vi "Omron TCP FINS-Command Frame.vi"(8 "error in":errorcluster, 10 "FINS Command Frame":T3, 11 "Buffer Data In":T1) -> (0 "error out":errorcluster, 3 "Buffer Data Out":T1)   [LabVIEW 2016]
uses:
  Data Def/Omron TCP FINS-FINS Command Frame.ctl
  Data Def/Omron TCP FINS-Command Code.ctl
  Data Def/Omron TCP FINS-Buffer Data.ctl
  Data Def/Omron TCP FINS-Memory Area Read Data.ctl
  Data Def/Omron TCP FINS-Memory Area Write Data.ctl
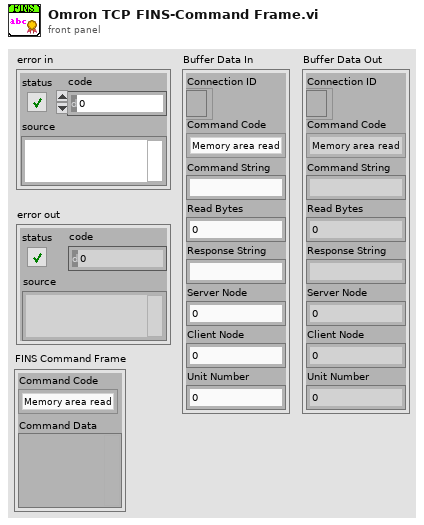
[diagram p1: front panel]
types:
  T1 = typedef "Omron TCP FINS-Buffer Data.ctl" = cluster{"Connection ID":refnum<k5>, "Command Code":T2, "Command String":string, "Read Bytes":i32, "Response String":string, "Server Node":u8, "Client Node":u8, "Unit Number":u8}
  T2 = typedef "Omron TCP FINS-Command Code.ctl" = enum16{"Memory area read", "Memory area write"}
  T3 = typedef "Omron TCP FINS-FINS Command Frame.ctl" = cluster{"Command Code":T2, "Command Data":variant}
  T4 = typedef "Omron TCP FINS-Memory Area Read Data.ctl" = cluster{"I/O Memory Address":u8, "Beginning Address":u16, "No. Of Items":u16}
  T5 = typedef "Omron TCP FINS-Memory Area Write Data.ctl" = cluster{"I/O Memory Address":u8, "Beginning Address":u16, "Data":i16[]}
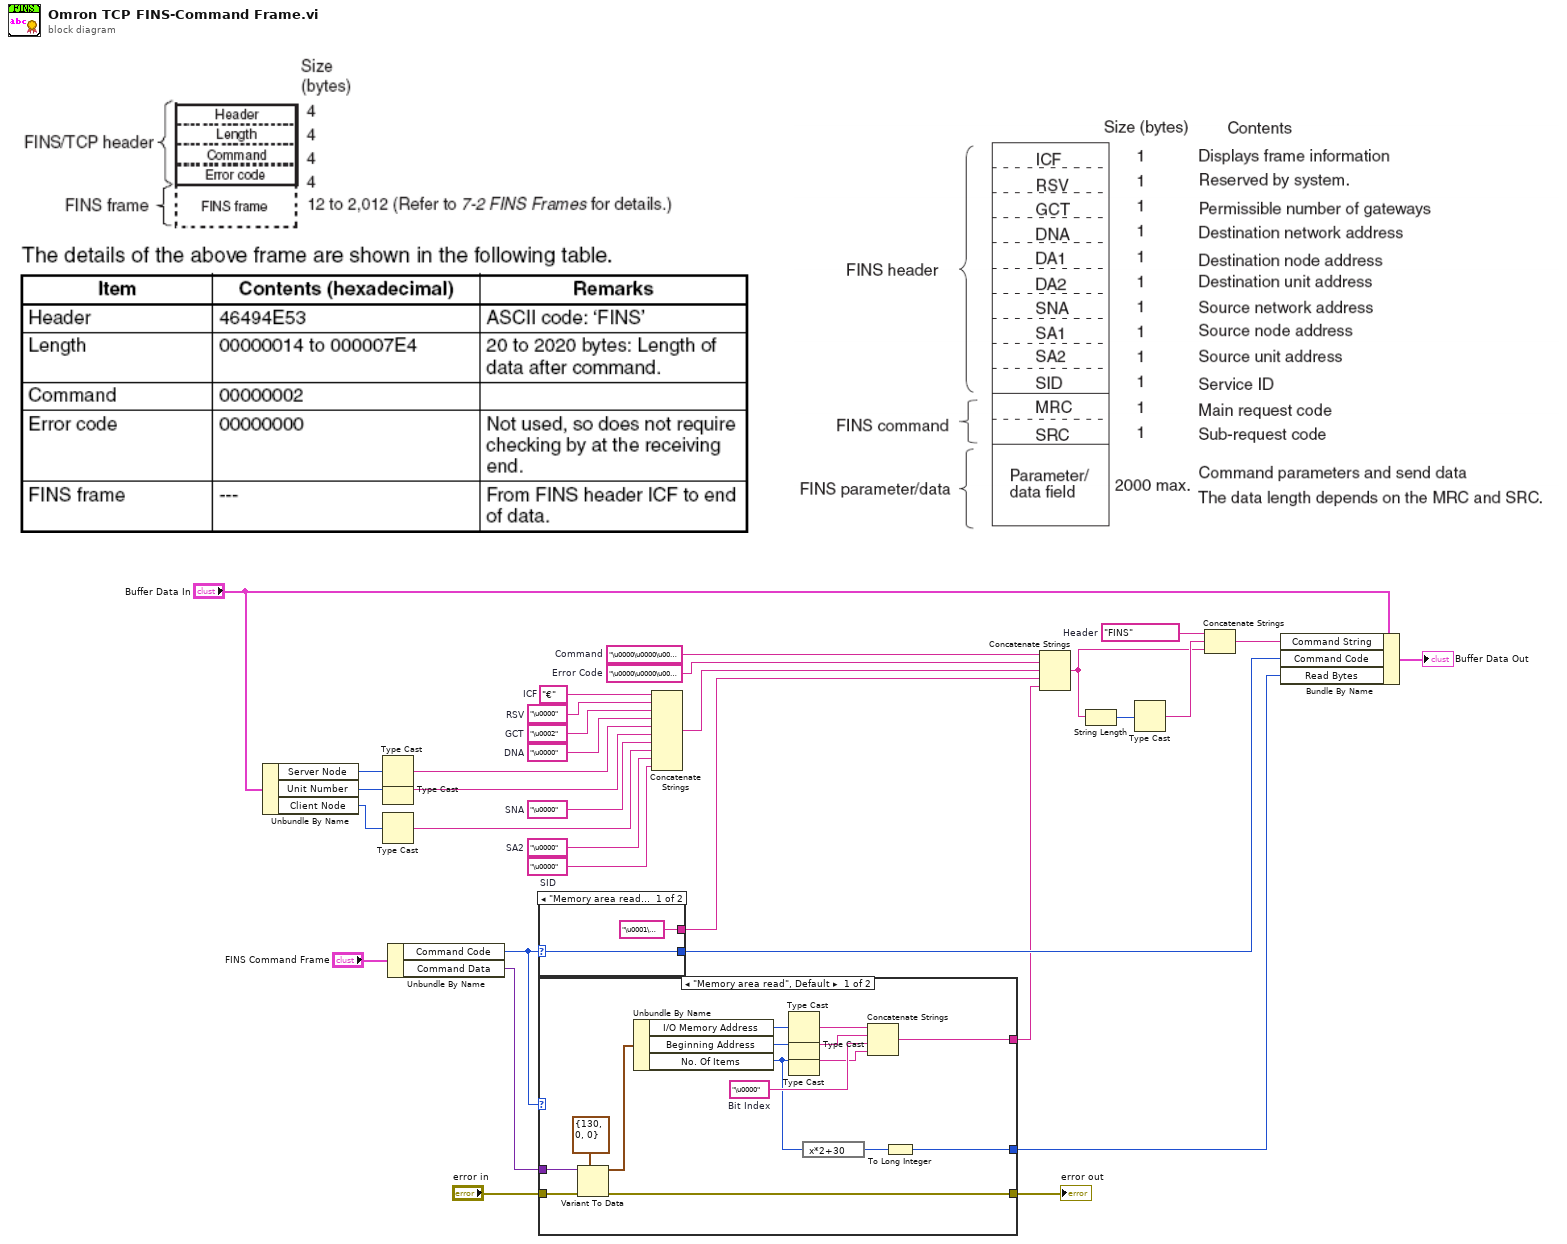
[diagram p0: block diagram]
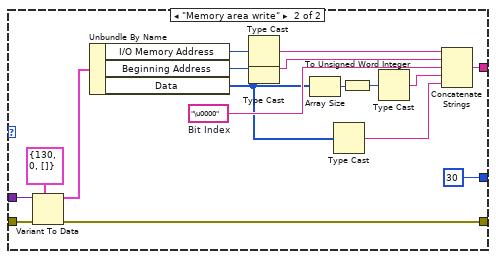
[diagram p2: hidden frame]
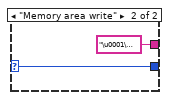
[diagram p3: hidden frame]
diagram:
  w18 = "\u0000\u0000\u0000\u0000"  # Error Code
  w19 = "\u0000\u0000\u0000\u0002"  # Command
  w20 = "\u0000"  # SID
  w21 = "\u0000"  # SA2
  w22 = "\u0000"  # SNA
  w23 = "\u0000"  # DNA
  w24 = "\u0002"  # GCT
  w25 = "\u0000"  # RSV
  w26 = "€"  # ICF
  w3 = "FINS"  # Header
  n1 = Unbundle By Name("Buffer Data In") -> ("Server Node"=w15:u8, "Unit Number"=w13:u8, "Client Node"=w11:u8)
  n2 = Type Cast(x=w15) -> (*(type *) &x=w14:string)  [unwired: 1 in]
  n3 = Type Cast(x=w13) -> (*(type *) &x=w12:string)  [unwired: 1 in]
  n4 = Type Cast(x=w11) -> (*(type *) &x=w10:string)  [unwired: 1 in]
  n5 = Unbundle By Name("FINS Command Frame") -> ("Command Code"=w32:T2, "Command Data"=w31:variant)
  n6 = case shown="\"Memory area read\", Default" w32 {
    selector: w32 -> [w33 w35]
    tunnel: ["\u0001\u0001" ("Command code") "\u0001\u0002" ("Command code")] -> w8
    tunnel: [w33 w35] -> w28
    frame "Memory area read", Default {
    }
    frame "Memory area write" {
    }
  }
  n7 = case shown="\"Memory area read\", Default" w32 {
    tunnel: w31 -> [w50 w67]
    tunnel: "error in" -> [w51 w68]
    tunnel: [w47 w65] -> w29
    tunnel: [w40 w64] -> w7
    tunnel: [w37 30 ("No. Of Items")] -> w27
    frame "Memory area read", Default {
      w42 = "\u0000"  # Bit Index
      n8 = Variant To Data(error in=w51, type=T4 {"I/O Memory Address"=130, "Beginning Address"=0, "No. Of Items"=0} ("Memory Area Read Data"), Variant=w50) -> (data=w48:T4, error out=w47:errorcluster)
      n9 = Unbundle By Name(w48) -> ("I/O Memory Address"=w46:u8, "Beginning Address"=w45:u16, "No. Of Items"=w39:u16)
      n10 = Type Cast(x=w46) -> (*(type *) &x=w44:string)  [unwired: 1 in]
      n11 = Type Cast(x=w45) -> (*(type *) &x=w43:string)  [unwired: 1 in]
      n12 = Type Cast(x=w39) -> (*(type *) &x=w41:string)  [unwired: 1 in]
      n13 = expression code="x*2+30"(w39) -> (w38:u16)
      n14 = Concatenate Strings(w44, w43, w42, w41) -> (w40:string)
      n15 = To Long Integer(number=w38) -> (32bit integer=w37:i32)
    }
    frame "Memory area write" {
      w57 = "\u0000"  # Bit Index
      n16 = Variant To Data(error in=w68, type=T5 {"I/O Memory Address"=130, "Beginning Address"=0, "Data"=[]} ("Memory Area Write Data"), Variant=w67) -> (data=w66:T5, error out=w65:errorcluster)
      n17 = Unbundle By Name(w66) -> ("I/O Memory Address"=w61:u8, "Beginning Address"=w60:u16, "Data"=w53:i16[])
      n18 = Type Cast(x=w61) -> (*(type *) &x=w59:string)  [unwired: 1 in]
      n19 = Type Cast(x=w60) -> (*(type *) &x=w58:string)  [unwired: 1 in]
      n20 = Array Size(array=w53) -> (size(s)=w56:i32)
      n21 = Type Cast(x=w53) -> (*(type *) &x=w52:string)  [unwired: 1 in]
      n22 = To Unsigned Word Integer(number=w56) -> (unsigned 16bit integer=w55:u16)
      n23 = Type Cast(x=w55) -> (*(type *) &x=w54:string)  [unwired: 1 in]
      n24 = Concatenate Strings(w59, w58, w57, w54, w52) -> (w64:string)
    }
  }
  "error out" <- w29
  n25 = Concatenate Strings(w26, w25, w24, w23, w14, w12, w22, w10, w21, w20) -> (w17:string)
  n26 = Concatenate Strings(w19, w18, w17, w8, w7) -> (w4:string)
  n27 = String Length(string=w4) -> (length=w6:i32)
  n28 = Type Cast(x=w6) -> (*(type *) &x=w5:string)  [unwired: 1 in]
  n29 = Concatenate Strings(w3, w5, w4) -> (w2:string)
  n30 = Bundle By Name(cluster="Buffer Data In", "Command String"=w2, "Command Code"=w28, "Read Bytes"=w27) -> (→"Buffer Data Out":T1)
